vi "SCXI-1141 Hardware Filtering.vi"() -> ()   [LabVIEW 2010]
panel:
  in  "DAQmx Task Name":refnum<k21>="FilterTask"
  in  "new values?":bool
  in  "Cutoff Freq":dbl=250.0
  in  "rate":dbl=10000.0 format="%0.2f"
  out "Power Spectrum":dynamicdata(graph)
  out "Waveform Graph":waveform(dbl)[](graph)
  in  "stop":bool
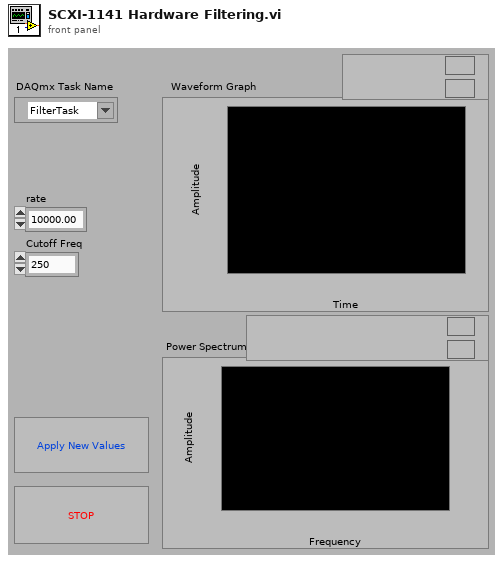
[diagram p1: front panel]
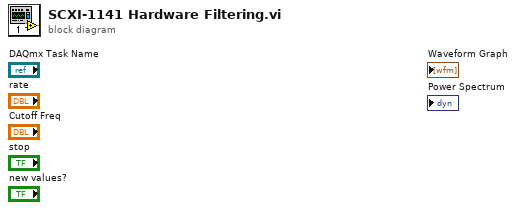
[diagram p0: block diagram]
diagram:
